vi "TEST SCREEN UPDATE _1.vi"(0 "Staion  in 1":refnum<k5>, 2 "Staion  in 2":refnum<k5>, 3 "Staion  in error 2":errorcluster, 4 "Staion  in 3":refnum<k5>, 5 "Staion  in error 3":errorcluster, 6 "DataBase connection in":T2, 7 "Database error in":errorcluster, 21 "Staion  in error 1":errorcluster) -> (1 "Staion Error Out 1":errorcluster, 20 "Staion Out 1":refnum<k5>, 22 "Staion Out 2":refnum<k5>, 23 "Staion Error Out 2":errorcluster, 24 "Staion Out 3":refnum<k5>, 25 "Staion Error Out 3":errorcluster, 26 "Database connection out":T2, 27 "Database error out":errorcluster)   [LabVIEW 2023]
uses:
  <vilib>/addons/database/Connection.llb/Conn ObjectReference.ctl
  Data base/database cluster.ctl
  test sequnece leak.ctl
  test setting.ctl
  Variable/Global.vi
  <vilib>/addons/database/NI_Database_API.lvlib
panel:
  out "STN 1 MSG":string caption="Scan Barcode"
  in  "Exit":bool
  in  "Tab Control":enum32{"main", "Other"}(tab)
  out "RESULT_ST_01":string="0" caption="RESULT"
  out "Weight(gm)":string="0"
  out "Torque(Nm)":string="0"
  out "Child Part 4":string caption="Batery Batchcode"
  out "Child Part 3":string
  out "Child Part 2":string
  out "Child Part 1":string
  out "STN 2 MSG":string caption="Scan Barcode"
  out "Result":string[][](table)
  out "Part Barcode":string
  in  "Tab Control 2":enum32{"station 1", "station 2", "station 3"}(tab)
  out "STN STR 1":string[](array[string])
  in  "Barcode OK":bool
  in  "Barcode NG":bool
  in  "Barcode Already":bool
  in  "M 1":T1
  out "STN  INTEGER_1":u16[][](array[numeric])
  out "STN FLOAT_1":sgl[][](array[numeric])
  in  "Barcode Already 2":bool
  in  "Barcode NG 2":bool
  in  "Barcode OK 2":bool
  in  "M 2":T1
  out "STN STR 2":string[](array[string])
  in  "M 3":T1
  in  "Barcode Already 3":bool
  in  "Barcode NG 3":bool
  in  "Barcode OK 3":bool
  out "STN STR 3":string[](array[string])
  out "sr. out BARCODE":i32
  out "sr. out Laser":i32
  out "length":i32
  out "Communication error 3":bool
  out "Communication error 2":bool
  out "Communication error 1":bool
  out "path for Laser sr":path
  out "path for Barcode sr.":path
  in  "Model NAME":string
  in  "count Path":path=path "D:/Configuration Folder Barcode/srno"
  in  "Visible":bool
  out "Exit 3":bool
  in  "TEST SETTING PATH":path=path "D:/Data Actuator/config/Settings"
  in  "Setting":path=path "D:/data/Test Settings"
  # "TESTING DATALOGGING SYSTEM"
  # "Test Screen"
  # "Station  10"
  # "Station 20"
  # "Station 30"
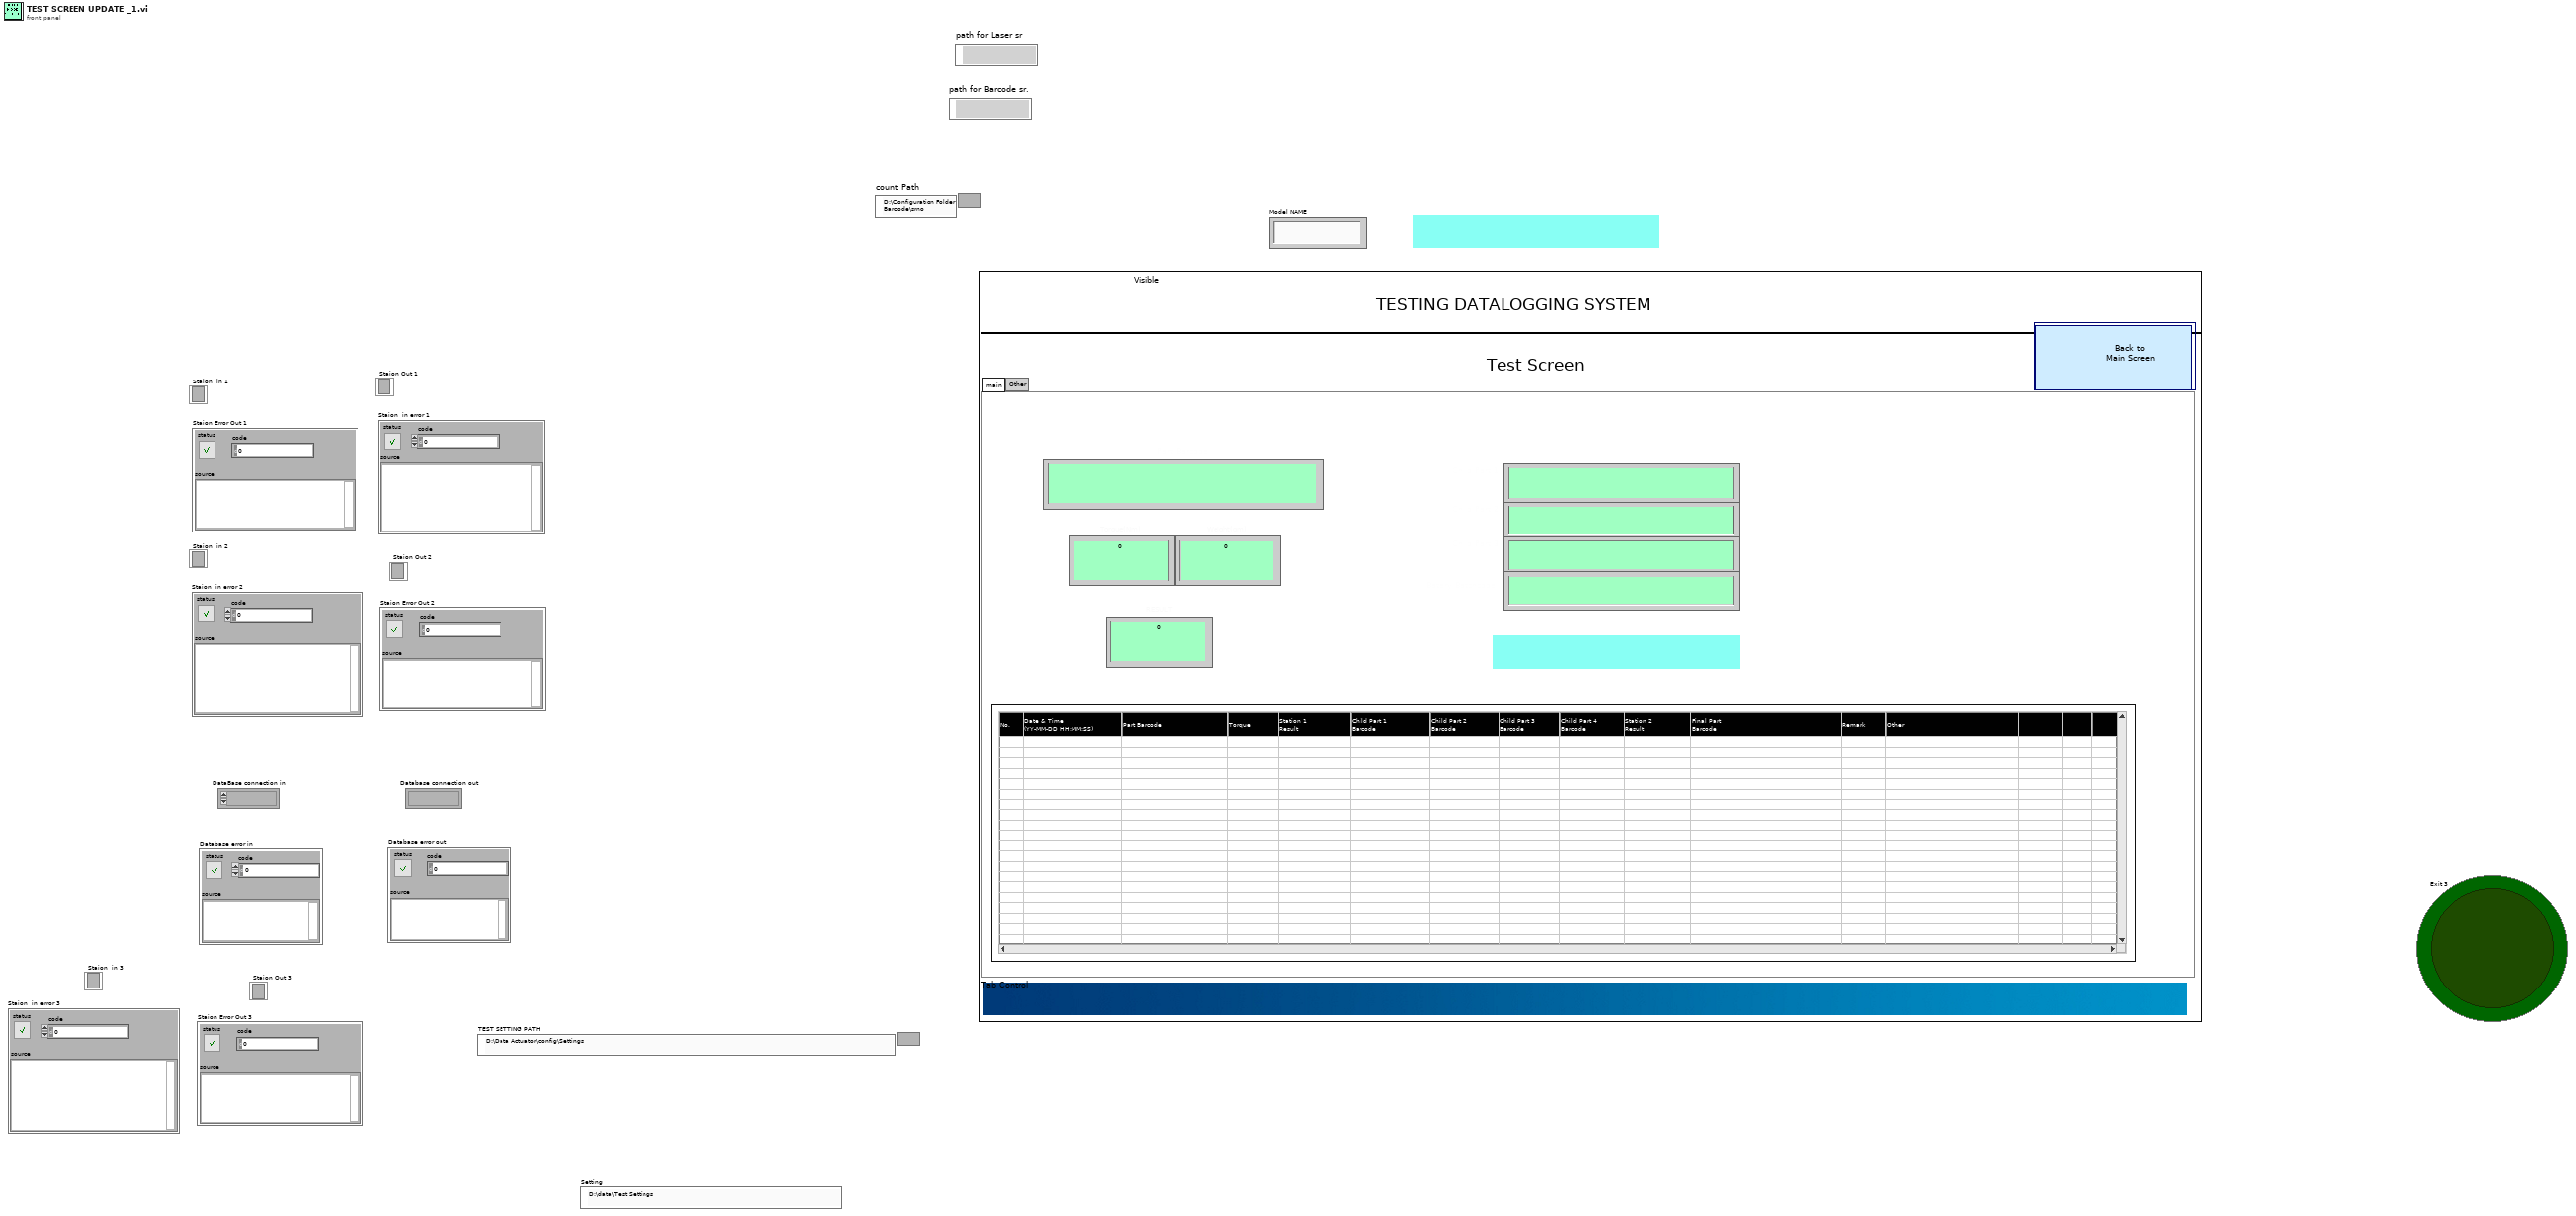
[diagram p1: front panel]
types:
  T1 = cluster{"Test Start Leak":bool, "Test Stop Leak":bool, "Scan Barcode":bool, "Test Running":bool, "Test OK":bool, "Test NG":bool, "Spare 1":bool, "Spare 2":bool}
  T2 = typedef "NI_Database_API.lvlib/Conn ObjectReference.ctl" = refnum<k1>
  T3 = typedef "database cluster.ctl" = cluster{"ID":i64, "Datetime":string, "PARTBARCODE":string, "TORQUE":string, "RESULT1":string, "CHILD1":string, "CHILD2":string, "CHILD3":string, "CHILD4":string, "RESULT2":string, "FINALBARCODE":string, "RESULT3":string, "REMARK":string, "OTHER":string}
  T4 = enum16{"open", "replace", "create", "open or create", "replace or create", "replace or create with confirmation"}
  T5 = typedef "test setting.ctl" = cluster{"M&M Part No.":string, "Vendor Code":string, "Part Identification Code":string, "Next Barcode Printing Wait Time":i32, "Path for LAser":path}
  T6 = typedef "test sequnece leak.ctl" = enum16{"Intilize", "CYCLE RESET", "Wait For teststart", "wait for scan", "check Barcode", "wait for start", "Wait for result", "wait for complete", "test stop", "Wait for LAser Scan Data", "check Scan Laser Data", "data save", "update tabel", "send data to Laser", "wait for Laser Start", "wait for laser stop"}
  T7 = typedef "Communication setting.ctl" = cluster{"Light Scanner Port":refnum<visa-resource-name>, "Shift-A":timestamp, "Shift-B":timestamp, "Shift-C":timestamp, "Leak Scanner Port":refnum<visa-resource-name>, "Barcode Printer":refnum<visa-resource-name>}
  T8 = cluster{"M--- 0-7[0]":bool, "M--- 0-7[1]":bool, "M--- 0-7[2]":bool, "M--- 0-7[3]":bool, "M--- 0-7[4]":bool, "M--- 0-7[5]":bool, "M--- 0-7[6]":bool, "M--- 0-7[7]":bool}
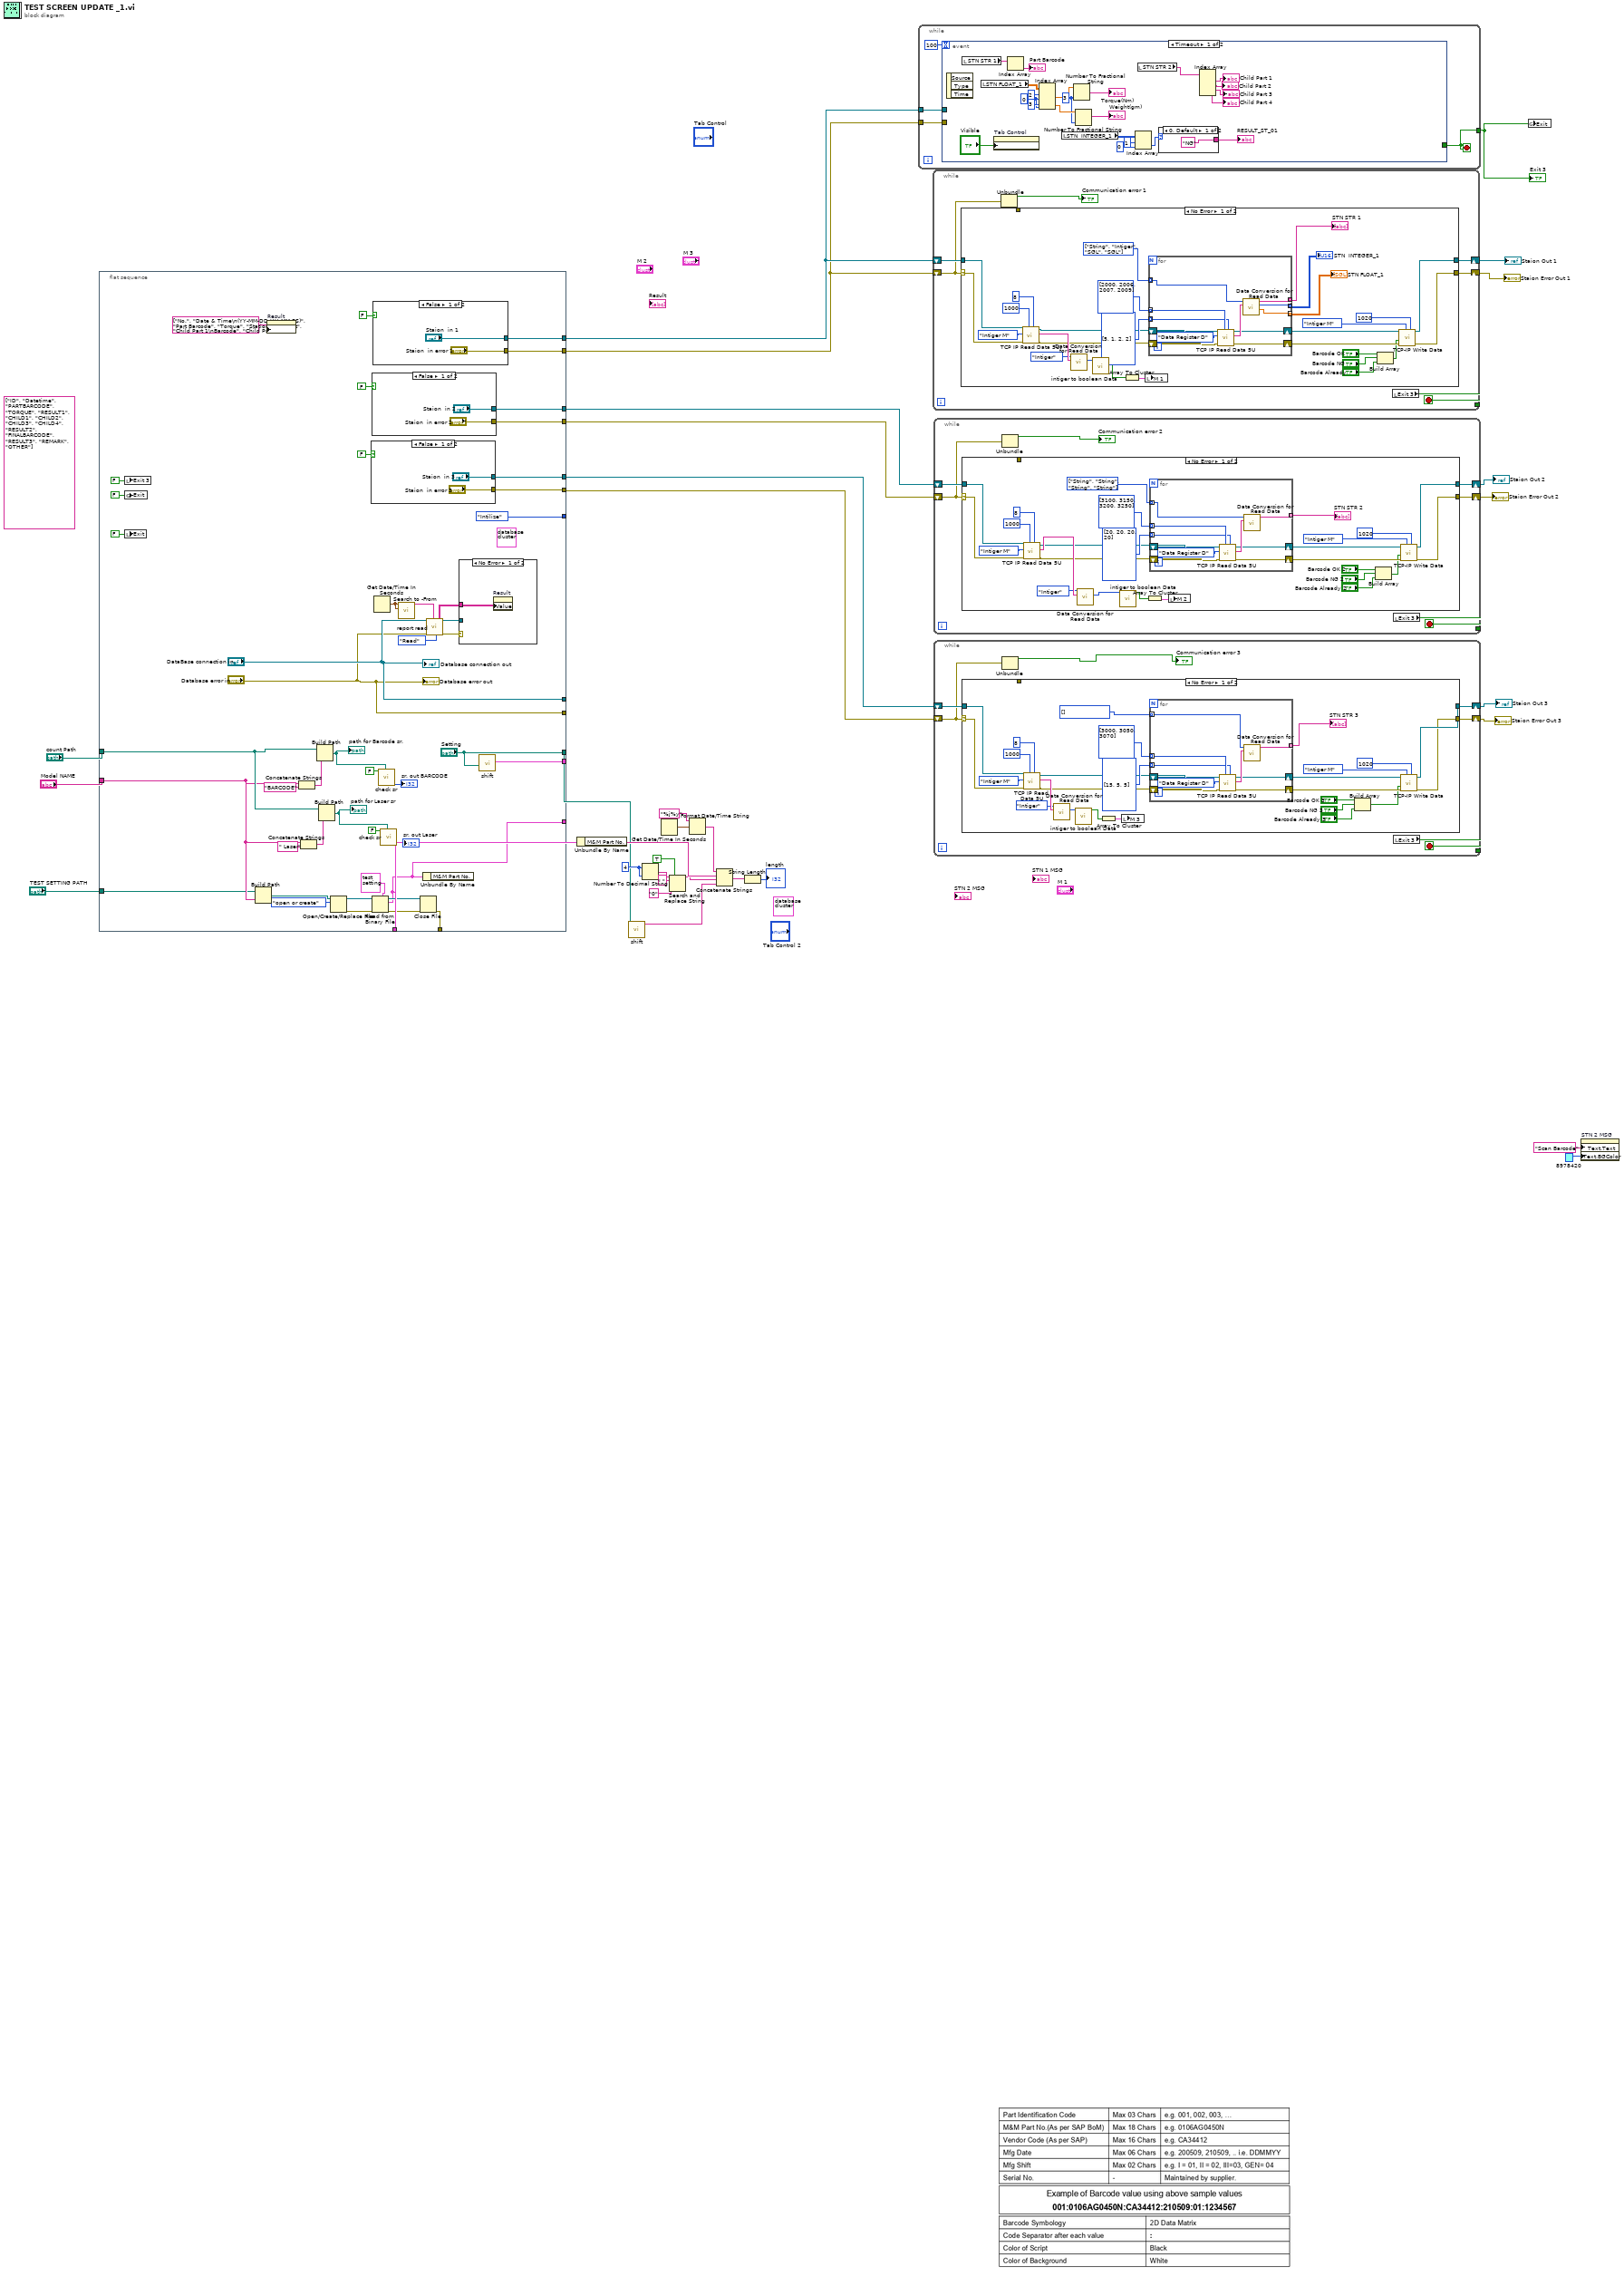
[diagram p0: block diagram]
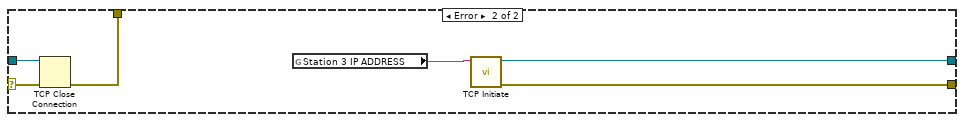
[diagram p2: hidden frame]
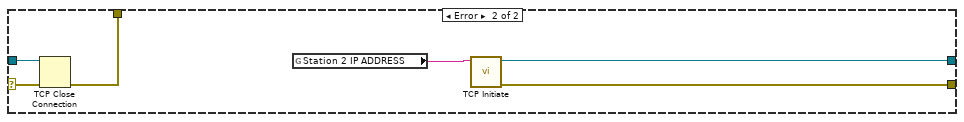
[diagram p3: hidden frame]
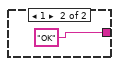
[diagram p4: hidden frame]
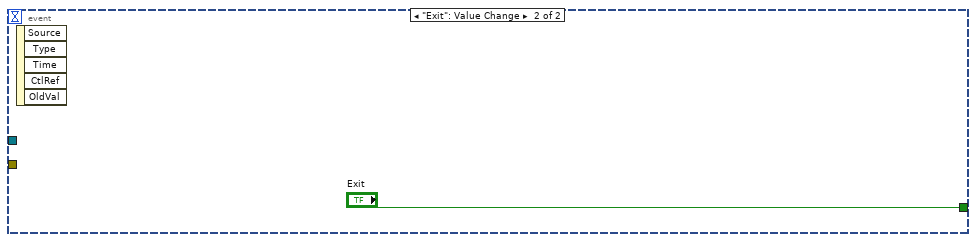
[diagram p5: hidden frame]
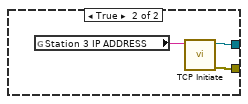
[diagram p6: hidden frame]
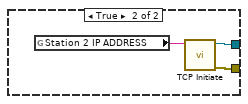
[diagram p8: hidden frame]
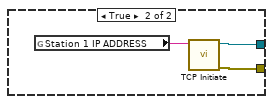
[diagram p9: hidden frame]
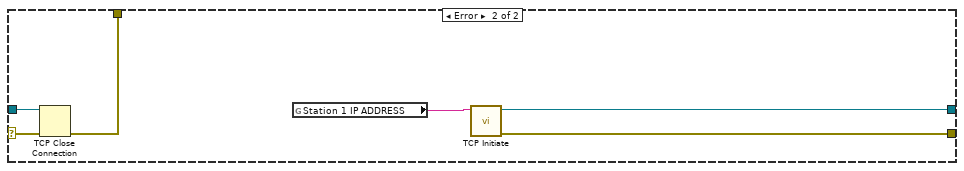
[diagram p10: hidden frame]
diagram:
  (unwired) string[] ["ID", "Datetime", "PARTBARCODE", "TORQUE", "RESULT1", "CHILD1", "CHILD2", "CHILD3", "CHILD4", "RESULT2", "FINALBARCODE", "RESULT3", "REMARK", "OTHER"] ("tables")
  w15 = i16 4 ("width (-)")
  (unwired) T3 {"ID"=0, "Datetime"="", "PARTBARCODE"="", "TORQUE"="", "RESULT1"="", "CHILD1"="", "CHILD2"="", "CHILD3"="", "CHILD4"="", "RESULT2"="", "FINALBARCODE"="", "RESULT3"="", "REMARK"="", "OTHER"=""} ("Data")
  n1 = flat-sequence {
    tunnel: ["Setting"] -> w14
    tunnel: [w78] -> _
    tunnel: [w76] -> w31
    tunnel: [w75] -> w30
    tunnel: [test_sequnece_leak."Intilize" ("Enum 2")] -> _
    tunnel: [w69] -> w6
    tunnel: [w68] -> w5
    tunnel: ["DataBase connection in"] -> _
    tunnel: ["Database error in"] -> _
    tunnel: [w55] -> _
    tunnel: [w37] -> _
    tunnel: "count Path" -> [w40]
    tunnel: "Model NAME" -> [w39]
    tunnel: "TEST SETTING PATH" -> [w38]
    tunnel: [w37] -> w16
    tunnel: [w35] -> w4
    tunnel: [w34] -> w3
    frame #0 {
      (unwired) T3 {"ID"=0, "Datetime"="", "PARTBARCODE"="", "TORQUE"="", "RESULT1"="", "CHILD1"="", "CHILD2"="", "CHILD3"="", "CHILD4"="", "RESULT2"="", "FINALBARCODE"="", "RESULT3"="", "REMARK"="", "OTHER"=""} ("Data")
      n2 = local write "Exit 3"(FALSE ("Exit 3")) -> ()
      n3 = global write "Global.vi" "Exit"(FALSE ("Exit")) -> ()
      n4 = local write "Exit"(FALSE ("Exit")) -> ()
      n5 = Build Path(base path=w38, name or relative path=w39) -> (appended path=w57:path)
      n6 = property on="Result" class="Tbl (strict)"("Column Headers[]"=string[] ["No.", "Date & Time\n(YY-MM-DD HH:MM:SS)", "Part Barcode", "Torque", "Station 1\nResult", "Child Part 1\nBarcode", "Child Part 2\nBarcode", "Child Part 3\nBarcode", "Child Part 4\nBarcode", "Station 2\nResult", "Final Part\nBarcode", "Remark", "Other"] ("Column Header Strings[]")) -> ()  [unwired: 2 in, 2 out]
      n7 = Concatenate Strings(w39, "BARCODE" ("string")) -> (w63:string)
      n8 = Concatenate Strings(w39, " Laser" ("string")) -> (w45:string)
      n9 = Build Path(base path=w40, name or relative path=w63) -> (appended path=w64:path)
      "path for Barcode sr." <- w64
      n10 = Build Path(base path=w40, name or relative path=w45) -> (appended path=w44:path)
      "path for Laser sr" <- w44
      n11 = Open/Create/Replace File(file path (use dialog)=w57, operation (0:open)=T4."open or create") -> (refnum out=w62:refnum<file>, error out=w61:errorcluster)  [unwired: 4 in, 1 out]
      n12 = case shown="False" FALSE {
        tunnel: ["Staion  in 3" w84] -> w35
        tunnel: ["Staion  in error 3" w83] -> w34
        frame False {
        }
        frame True {
          n13 = global read "Global.vi" "Station 3 IP ADDRESS"() -> (w82:string)
          n14 = call "TCP Initiate.vi"("IP ADDRESS"=w82) -> ("error out"=w83:errorcluster, "connection ID"=w84:refnum<k5>)  [unwired: 9 in]
        }
      }
      n15 = case shown="False" FALSE {
        tunnel: ["Staion  in 2" w90] -> w69
        tunnel: ["Staion  in error 2" w89] -> w68
        frame False {
        }
        frame True {
          n16 = global read "Global.vi" "Station 2 IP ADDRESS"() -> (w88:string)
          n17 = call "TCP Initiate.vi"("IP ADDRESS"=w88) -> ("error out"=w89:errorcluster, "connection ID"=w90:refnum<k5>)  [unwired: 9 in]
        }
      }
      n18 = Read from Binary File(5:T5 {"M&M Part No."="", "Vendor Code"="02BHMSI1009190338RKWPG", "Part Identification Code"="02CRMTT1009190250KWPG", "Next Barcode Printing Wait Time"=0, "Path for LAser"=path ""} ("Cluster"), 8:w61, 11:w62) -> (0:w60:errorcluster, 2:w37:T5, 3:w59:refnum<file>)  [unwired: 3 in, 1 out]
      n19 = case shown="False" FALSE {
        tunnel: ["Staion  in 1" w95] -> w76
        tunnel: ["Staion  in error 1" w94] -> w75
        frame False {
        }
        frame True {
          n20 = global read "Global.vi" "Station 1 IP ADDRESS"() -> (w93:string)
          n21 = call "TCP Initiate.vi"("IP ADDRESS"=w93) -> ("error out"=w94:errorcluster, "connection ID"=w95:refnum<k5>)  [unwired: 9 in]
        }
      }
      n22 = Get Date/Time In Seconds() -> (seconds since 1Jan1904=w54:timestamp)
      n23 = call "check sr.vi"("file path (use dialog)"=w64, "writeL:t"=FALSE) -> ("sr. out"=→"sr. out BARCODE":i32)  [unwired: 9 in]
      n24 = call "check sr.vi"("file path (use dialog)"=w44, "writeL:t"=FALSE) -> ("sr. out"=→"sr. out Laser":i32)  [unwired: 9 in]
      n25 = call "Search to -From.vi"("From date"=w54, "To Date"=w54) -> ("search dataString"=w51:string)  [unwired: 9 in]
      n26 = Close File(refnum=w59, error in=w60) -> (error out=w55:errorcluster)  [unwired: 1 out]
      n27 = Unbundle By Name(w37) -> ()  [unwired: 1 out]
      n28 = call "report read.vi"("connection reference"="DataBase connection in", "error in (no error)"="Database error in", "search dataString"=w51, "Enum"=enum16{"Write", "Read"}."Read") -> ("Search Reverse"=w50:string[][], "connection reference out"=w49:T2, "error out"=w52:errorcluster)  [unwired: 10 in, 3 out]
      n29 = case shown="No Error" w52 {
        tunnel: w50 -> [w85 _]
        tunnel: w49 -> [_ _]
        frame No Error {
          n30 = property on="Result" class="Tbl (strict)"("Value"=w85) -> ()  [unwired: 2 in, 2 out]
        }
        frame Error {
        }
      }
      n31 = call "shift.vi"("Setting"="Setting") -> ("data"=w78:T7)  [unwired: 9 in, 1 out]
      "Database connection out" <- "DataBase connection in"
      "Database error out" <- "Database error in"
    }
  }
  n32 = Unbundle By Name(w16) -> ("M&M Part No."=w25:string)
  n33 = call "shift.vi"("Setting"=w14) -> ("SHIFT_A"=w13:string)  [unwired: 9 in, 1 out]
  n34 = Number To Decimal String(number=w15, width (-)=w15) -> (decimal integer string=w17:string)
  n35 = Get Date/Time In Seconds() -> (seconds since 1Jan1904=w21:timestamp)
  n36 = Search and Replace String(replace all?=TRUE ("replace all? (F)"), input string=w17, search string=" ", replace string="0" ("replace string (\"\")")) -> (result string=w20:string)  [unwired: 4 in, 3 out]
  n37 = Format Date/Time String(time format string (%c)="%j%y", seconds (now)=w21) -> (date/time string=w24:string)  [unwired: 1 in]
  n38 = Concatenate Strings(w24, w25, w20, w13) -> (w12:string)
  n39 = String Length(string=w12) -> (length=→"length":i32)
  n40 = while {
    tunnel: w31 -> [w98]
    tunnel: w30 -> [w97]
    tunnel: [w96] -> w29
    stop <- w96 stop-if-true
    n41 = event shown="[0] Timeout" {
      selector: _ -> [_ _]
      dyn-events: _ -> [_ _]
      timeout: 100 -> [_ _]
      tunnel: [_ "Exit"] -> w96
      tunnel: w98 -> [_ _]
      tunnel: w97 -> [_ _]
      event Timeout {
        w111 = i16 3 ("precision (6)")
        w115 = 0 ("disabled index (col)")
        n42 = event-data() -> ()  [unwired: 1 in, 3 out]
        n43 = local read "STN STR 1"() -> (w119:string[])
        n44 = local read "STN FLOAT_1"() -> (w118:sgl[][])
        n45 = property on="Tab Control" class="TabCtl (strict)"("Page Labels Display Visible?"="Visible") -> ()  [unwired: 2 in, 2 out]
        n46 = Index Array(array=w119) -> (element=→"Part Barcode":string)  [unwired: 1 in]
        n47 = Index Array(array=w118, index (row) #1=2 ("index (row)"), index (col) #1=w115, index (row) #2=3 ("index (row)"), index (col) #2=w115) -> (element #1=w114:sgl, element #2=w112:sgl)
        n48 = local read "STN  INTEGER_1"() -> (w104:u16[][])
        n49 = Number To Fractional String(number=w114, precision (6)=w111) -> (F-format string=→"Torque(Nm)":string)  [unwired: 2 in]
        n50 = Number To Fractional String(number=w112, precision (6)=w111) -> (F-format string=→"Weight(gm)":string)  [unwired: 2 in]
        n51 = Index Array(array=w104, index (row)=1, index (col)=0 ("disabled index (col)")) -> (element=w102:u16)
        n52 = local read "STN STR 2"() -> (w109:string[])
        n53 = case shown="0, Default" w102 {
          tunnel: ["NG" ("RESULT_ST_01") "OK" ("RESULT_ST_01")] -> w100
          frame 0, Default {
          }
          frame 1 {
          }
        }
        "RESULT_ST_01" <- w100
        n54 = Index Array(array=w109) -> (element #1=→"Child Part 1":string, element #2=→"Child Part 2":string, element #3=→"Child Part 3":string, element #4=→"Child Part 4":string)  [unwired: 4 in]
      }
      event "Exit": Value Change {
        n55 = event-data() -> ()  [unwired: 1 in, 5 out]
      }
    }
  }
  "Exit 3" <- w29
  n56 = while {
    tunnel: [w126] -> _
    shift-right: [w130] -> w33
    shift-left: w31 -> [w129]
    shift-right: [w128] -> w32
    shift-left: w30 -> [w127]
    stop <- w126 stop-if-true
    n57 = case shown="No Error" w127 {
      selector: w127 -> [w151 w174]
      tunnel: [w139 w176] -> w130
      tunnel: [w138 w175] -> w128
      tunnel: w129 -> [w152 w173]
      tunnel: [_ w172] -> _
      frame No Error {
        w133 = enum16{"String", "Intiger", "DBL", "SGL"}[] [enum."String", enum."Intiger", enum."SGL", enum."SGL"] items=["String", "Intiger", "DBL", "SGL"]
        n58 = call "TCP IP Read Data 5U.vi"("No of data regiter read"=8, "Start Address"=1000, "error in"=w151, "Data Rigister/Memory"=enum16{"Data Register D", "Intiger M"}."Intiger M", "connection ID"=w152) -> ("error out"=w140:errorcluster, "RAw Data"=w157:string, "connection ID Out"=w141:refnum<k5>)  [unwired: 4 in]
        n59 = call "Data Conversion for Read Data.vi"("data out"=w157, "Read Data Type"=enum16{"String", "Intiger", "DBL"}."Intiger") -> ("M Intiger"=w158:u16[])  [unwired: 6 in, 3 out]
        n60 = call "intiger to boolean Data.vi"("data"=w158) -> ("M--- 0-7"=w136:bool[])  [unwired: 9 in, 5 out]
        n61 = Array To Cluster(array=w136) -> (cluster=w135:T8)
        n62 = local write "M 1"(w135) -> ()
        n63 = for {
          tunnel: [w164] -> w131 mode=indexing
          shift-right: [w166] -> w150
          shift-left: w141 -> [w168]
          shift-right: [w165] -> w149
          shift-left: w140 -> [w167]
          tunnel: i32[] [2000, 2006, 2007, 2009] -> [w163] mode=indexing
          tunnel: i32[] [5, 1, 2, 2] ("No of data regiter read") -> [w162] mode=indexing
          tunnel: [w161] -> w132 mode=indexing
          tunnel: [w160] -> w134 mode=indexing
          tunnel: w133 -> [w159] mode=indexing
          n64 = call "TCP IP Read Data 5U.vi"("No of data regiter read"=w162, "Start Address"=w163, "error in"=w167, "Data Rigister/Memory"=enum16{"Data Register D", "Intiger M"}."Data Register D", "connection ID"=w168) -> ("error out"=w165:errorcluster, "RAw Data"=w169:string, "connection ID Out"=w166:refnum<k5>)  [unwired: 4 in]
          n65 = call "Data Conversion for Read Data.vi"("data out"=w169, "Read Data Type"=w159) -> ("Data regiter"=w161:sgl[], "M Intiger"=w160:u16[], "String"=w164:string)  [unwired: 6 in, 1 out]
        }
        "STN STR 1" <- w131
        "STN  INTEGER_1" <- w134
        "STN FLOAT_1" <- w132
        n66 = Build Array("Barcode OK", "Barcode NG", "Barcode Already") -> (w147:bool[])
        n67 = call "TCP-IP Write Data.vi"("Start address"=1020, "Data Rigister/Memory"=enum16{"Data Register D", "Intiger M"}."Intiger M", "error in (no error)"=w149, "M 16 bit Only"=w147, "connection ID"=w150) -> ("error out"=w138:errorcluster, "connection ID out"=w139:refnum<k5>)  [unwired: 5 in]
      }
      frame Error {
        n68 = TCP Close Connection(connection ID=w173, error in (no error)=w174) -> (error out=w172:errorcluster)  [unwired: 1 in, 1 out]
        n69 = global read "Global.vi" "Station 1 IP ADDRESS"() -> (w171:string)
        n70 = call "TCP Initiate.vi"("IP ADDRESS"=w171) -> ("error out"=w175:errorcluster, "connection ID"=w176:refnum<k5>)  [unwired: 9 in]
      }
    }
    n71 = Unbundle(w127) -> ("status"=→"Communication error 1":bool)  [unwired: 2 out]
    n72 = local read "Exit 3"() -> (w126:bool)
  }
  "Staion Out 1" <- w33
  "Staion Error Out 1" <- w32
  n73 = while {
    tunnel: [w178] -> _
    shift-right: [w182] -> w8
    shift-left: w6 -> [w181]
    shift-right: [w180] -> w7
    shift-left: w5 -> [w179]
    stop <- w178 stop-if-true
    n74 = case shown="No Error" w179 {
      selector: w179 -> [w201 w222]
      tunnel: [w189 w224] -> w182
      tunnel: [w188 w223] -> w180
      tunnel: w181 -> [w202 w221]
      tunnel: [_ w220] -> _
      frame No Error {
        w184 = enum16{"String", "Intiger", "DBL", "SGL"}[] [enum."String", enum."String", enum."String", enum."String"] items=["String", "Intiger", "DBL", "SGL"]
        n75 = call "TCP IP Read Data 5U.vi"("No of data regiter read"=8, "Start Address"=1000, "error in"=w201, "Data Rigister/Memory"=enum16{"Data Register D", "Intiger M"}."Intiger M", "connection ID"=w202) -> ("error out"=w190:errorcluster, "RAw Data"=w207:string, "connection ID Out"=w191:refnum<k5>)  [unwired: 4 in]
        n76 = call "Data Conversion for Read Data.vi"("data out"=w207, "Read Data Type"=enum16{"String", "Intiger", "DBL"}."Intiger") -> ("M Intiger"=w208:u16[])  [unwired: 6 in, 3 out]
        n77 = call "intiger to boolean Data.vi"("data"=w208) -> ("M--- 0-7"=w186:bool[])  [unwired: 9 in, 5 out]
        n78 = Array To Cluster(array=w186) -> (cluster=w185:T8)
        n79 = for {
          tunnel: [w212] -> w183 mode=indexing
          shift-right: [w214] -> w200
          shift-left: w191 -> [w216]
          shift-right: [w213] -> w199
          shift-left: w190 -> [w215]
          tunnel: i32[] [3100, 3150, 3200, 3250] -> [w211] mode=indexing
          tunnel: i32[] [20, 20, 20, 20] ("No of data regiter read") -> [w210] mode=indexing
          tunnel: w184 -> [w209] mode=indexing
          n80 = call "TCP IP Read Data 5U.vi"("No of data regiter read"=w210, "Start Address"=w211, "error in"=w215, "Data Rigister/Memory"=enum16{"Data Register D", "Intiger M"}."Data Register D", "connection ID"=w216) -> ("error out"=w213:errorcluster, "RAw Data"=w217:string, "connection ID Out"=w214:refnum<k5>)  [unwired: 4 in]
          n81 = call "Data Conversion for Read Data.vi"("data out"=w217, "Read Data Type"=w209) -> ("String"=w212:string)  [unwired: 6 in, 3 out]
        }
        "STN STR 2" <- w183
        n82 = local write "M 2"(w185) -> ()
        n83 = Build Array("Barcode OK 2", "Barcode NG 2", "Barcode Already 2") -> (w197:bool[])
        n84 = call "TCP-IP Write Data.vi"("Start address"=1020, "Data Rigister/Memory"=enum16{"Data Register D", "Intiger M"}."Intiger M", "error in (no error)"=w199, "M 16 bit Only"=w197, "connection ID"=w200) -> ("error out"=w188:errorcluster, "connection ID out"=w189:refnum<k5>)  [unwired: 5 in]
      }
      frame Error {
        n85 = TCP Close Connection(connection ID=w221, error in (no error)=w222) -> (error out=w220:errorcluster)  [unwired: 1 in, 1 out]
        n86 = global read "Global.vi" "Station 2 IP ADDRESS"() -> (w219:string)
        n87 = call "TCP Initiate.vi"("IP ADDRESS"=w219) -> ("error out"=w223:errorcluster, "connection ID"=w224:refnum<k5>)  [unwired: 9 in]
      }
    }
    n88 = Unbundle(w179) -> ("status"=→"Communication error 2":bool)  [unwired: 2 out]
    n89 = local read "Exit 3"() -> (w178:bool)
  }
  "Staion Out 2" <- w8
  "Staion Error Out 2" <- w7
  n90 = while {
    tunnel: [w226] -> _
    shift-right: [w230] -> w2
    shift-left: w4 -> [w229]
    shift-right: [w228] -> w1
    shift-left: w3 -> [w227]
    stop <- w226 stop-if-true
    n91 = case shown="No Error" w227 {
      selector: w227 -> [w249 w270]
      tunnel: [w237 w272] -> w230
      tunnel: [w236 w271] -> w228
      tunnel: w229 -> [w250 w269]
      tunnel: [_ w268] -> _
      frame No Error {
        w231 = enum16{"String", "Intiger", "DBL", "SGL"}[] [] items=["String", "Intiger", "DBL", "SGL"]
        n92 = call "TCP IP Read Data 5U.vi"("No of data regiter read"=8, "Start Address"=1000, "error in"=w249, "Data Rigister/Memory"=enum16{"Data Register D", "Intiger M"}."Intiger M", "connection ID"=w250) -> ("error out"=w238:errorcluster, "RAw Data"=w255:string, "connection ID Out"=w239:refnum<k5>)  [unwired: 4 in]
        n93 = call "Data Conversion for Read Data.vi"("data out"=w255, "Read Data Type"=enum16{"String", "Intiger", "DBL"}."Intiger") -> ("M Intiger"=w256:u16[])  [unwired: 6 in, 3 out]
        n94 = call "intiger to boolean Data.vi"("data"=w256) -> ("M--- 0-7"=w234:bool[])  [unwired: 9 in, 5 out]
        n95 = Array To Cluster(array=w234) -> (cluster=w233:T8)
        n96 = local write "M 3"(w233) -> ()
        n97 = for {
          tunnel: [w260] -> w232 mode=indexing
          shift-right: [w262] -> w248
          shift-left: w239 -> [w264]
          shift-right: [w261] -> w247
          shift-left: w238 -> [w263]
          tunnel: i32[] [3000, 3050, 3070] -> [w259] mode=indexing
          tunnel: i32[] [15, 5, 5] ("No of data regiter read") -> [w258] mode=indexing
          tunnel: w231 -> [w257] mode=indexing
          n98 = call "TCP IP Read Data 5U.vi"("No of data regiter read"=w258, "Start Address"=w259, "error in"=w263, "Data Rigister/Memory"=enum16{"Data Register D", "Intiger M"}."Data Register D", "connection ID"=w264) -> ("error out"=w261:errorcluster, "RAw Data"=w265:string, "connection ID Out"=w262:refnum<k5>)  [unwired: 4 in]
          n99 = call "Data Conversion for Read Data.vi"("data out"=w265, "Read Data Type"=w257) -> ("String"=w260:string)  [unwired: 6 in, 3 out]
        }
        "STN STR 3" <- w232
        n100 = Build Array("Barcode OK 3", "Barcode NG 3", "Barcode Already 3") -> (w245:bool[])
        n101 = call "TCP-IP Write Data.vi"("Start address"=1020, "Data Rigister/Memory"=enum16{"Data Register D", "Intiger M"}."Intiger M", "error in (no error)"=w247, "M 16 bit Only"=w245, "connection ID"=w248) -> ("error out"=w236:errorcluster, "connection ID out"=w237:refnum<k5>)  [unwired: 5 in]
      }
      frame Error {
        n102 = TCP Close Connection(connection ID=w269, error in (no error)=w270) -> (error out=w268:errorcluster)  [unwired: 1 in, 1 out]
        n103 = global read "Global.vi" "Station 3 IP ADDRESS"() -> (w267:string)
        n104 = call "TCP Initiate.vi"("IP ADDRESS"=w267) -> ("error out"=w271:errorcluster, "connection ID"=w272:refnum<k5>)  [unwired: 9 in]
      }
    }
    n105 = Unbundle(w227) -> ("status"=→"Communication error 3":bool)  [unwired: 2 out]
    n106 = local read "Exit 3"() -> (w226:bool)
  }
  "Staion Out 3" <- w2
  "Staion Error Out 3" <- w1
  n107 = global write "Global.vi" "Exit"(w29) -> ()
  n108 = property on="STN 2 MSG" class="Str"("Text.Text"="Scan Barcode", "Text.BGColor"=u32 8978420) -> ()  [unwired: 2 in, 2 out]
